vi "Email_Text_Files.vi"(0 "Filenames":path[](array[path]), 1 "message":string, 2 "subject ([No Subject])":string="[No Subject]") -> ()   [LabVIEW 2020]
uses:
  Email_transfer_global.vi
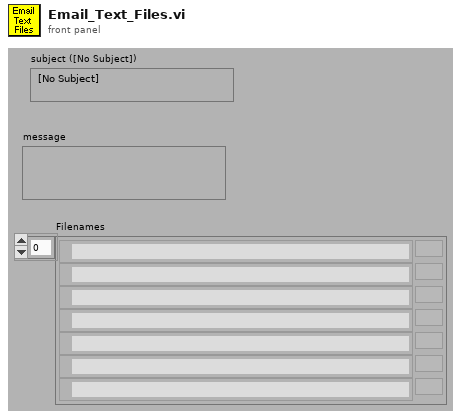
[diagram p1: front panel]
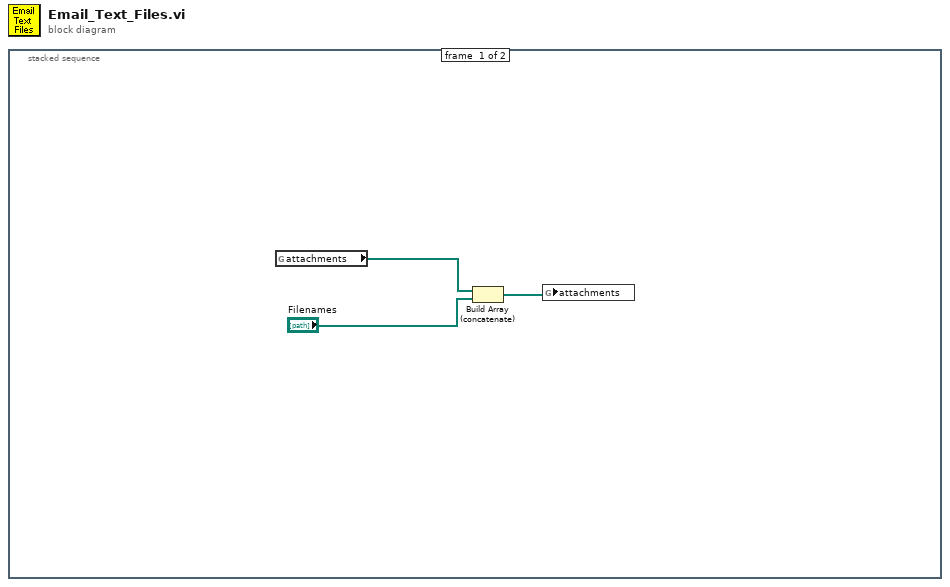
[diagram p0: block diagram]
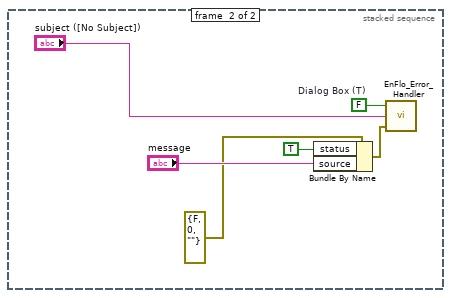
[diagram p2: hidden frame]
diagram:
  n1 = stacked-sequence {
    frame #0 {
      n2 = global read "Email_transfer_global.vi" "attachments"() -> (w3:path[])
      n3 = Build Array (concatenate)(w3, "Filenames") -> (w1:path[])
      n4 = global write "Email_transfer_global.vi" "attachments"(w1) -> ()
    }
    frame #1 {
      w9 = FALSE  # Dialog Box (T)
      n5 = Bundle By Name(cluster=errorcluster {"status"=FALSE, "code"=0, "source"=""} ("error in (no error)"), "status"=TRUE, "source"="message") -> (w6:errorcluster)
      n6 = call "EnFlo_Error_Handler.vi"("error in (no error)"=w6, "Error Type"="subject ([No Subject])", "Dialog Box (F)"=w9) -> ()  [unwired: 3 out]
    }
  }
